vi "Delete EngineLib from Target.vi"(7 "Library Name":string="Engine.lvlib", 8 "error in (no error)":errorcluster, 10 "Target Names in":string[](array[string]), 11 "Project Sync Tools in":refnum<class "Project Sync Tools.lvclass">) -> (0 "error out":errorcluster, 2 "Target Names out":string[](array[string]), 3 "Project Sync Tools out":refnum<class "Project Sync Tools.lvclass">)   [LabVIEW 2019, in "Project Sync Tools.lvclass"]
uses:
  Project Sync Tools.lvclass
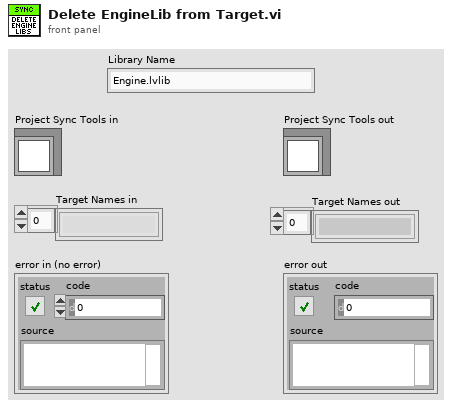
[diagram p1: front panel]
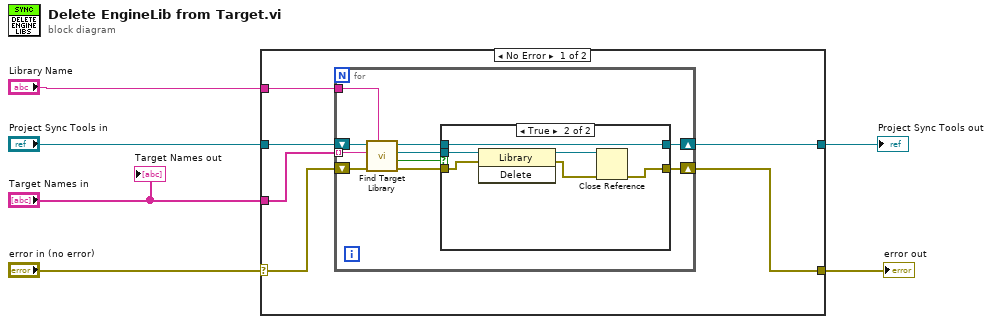
[diagram p0: block diagram]
diagram:
  n1 = case shown="No Error" "error in (no error)" {
    selector: "error in (no error)" -> [w8 w31]
    tunnel: [w12 w31] -> w6
    tunnel: [w11 w32] -> w5
    tunnel: "Target Names in" -> [w10 _]
    tunnel: "Project Sync Tools in" -> [w9 w32]
    tunnel: "Library Name" -> [w7 _]
    frame No Error {
      n2 = for {
        tunnel: w10 -> [w20] mode=indexing
        shift-right: [w14] -> w11
        shift-left: w9 -> [w22]
        shift-right: [w16] -> w12
        shift-left: w8 -> [w21]
        tunnel: w7 -> [w13]
        n3 = call "Find Target Library.vi"("Library Name"=w13, "error in (no error)"=w21, "Target Name"=w20, "CD Build Tools in"=w22) -> ("error out"=w18:errorcluster, "Found ?"=w19:bool, "Library out"=w17:refnum<vi>, "CD Build Tools out"=w15:refnum<class "Project Sync Tools.lvclass">)  [unwired: 4 in]
        n4 = case shown="True" w19 {
          tunnel: w18 -> [w24 w29]
          tunnel: w17 -> [_ w30]
          tunnel: [w24 w26] -> w16
          tunnel: w15 -> [w23 w25]
          tunnel: [w23 w25] -> w14
          frame False {
          }
          frame True {
            n5 = invoke class="Library" method="Delete"(reference=w30, error in=w29) -> (reference out=w27:refnum<vi>, error out=w28:errorcluster)  [unwired: 1 in, 1 out]
            n6 = Close Reference(reference=w27, error in (no error)=w28) -> (error out=w26:errorcluster)
          }
        }
      }
    }
    frame Error {
    }
  }
  "error out" <- w6
  "Project Sync Tools out" <- w5
  "Target Names out" <- "Target Names in"
